vi "RPI_PICO_example.vi"() -> ()   [LabVIEW 2020]
uses:
  <vilib>/Instr/_visa.llb/VISA Configure Serial Port (Instr).vi
panel:
  out "return count 2":u32
  out "VISA resource name out 2":refnum<visa-resource-name>
  out "readBuffer":string
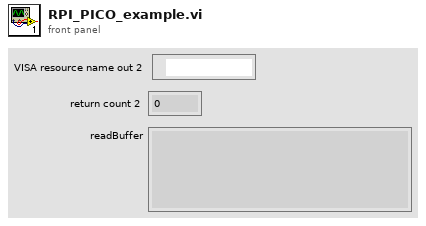
[diagram p1: front panel]
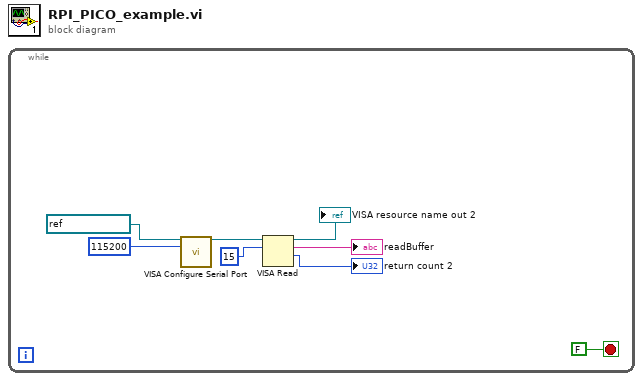
[diagram p0: block diagram]
diagram:
  n1 = while {
    stop <- FALSE stop-if-true
    n2 = call-poly "VISA Configure Serial Port"("VISA resource name"=refnum<visa-resource-name> "COM28", "baud rate (9600)"=u32 115200) -> ("VISA resource name out"=w7:refnum<visa-resource-name>)  [unwired: 12 in, 1 out]
    n3 = VISA Read(VISA resource name=w7, byte count=u32 15) -> (VISA resource name out=→"VISA resource name out 2":refnum<visa-resource-name>, read buffer=→"readBuffer":string, return count=→"return count 2":u32)  [unwired: 1 in, 1 out]
  }
